vi "Write Call Chain.vi"(10 "Call Chain":string[](array[string]), 11 "Assert in":refnum<class "Assert.lvclass">) -> (3 "Assert out":refnum<class "Assert.lvclass">)   [LabVIEW 2013, in "Caraya.lvlib" / "Assert.lvclass"]
uses:
  Assert.lvclass
  Assert.lvclass/Assert.ctl
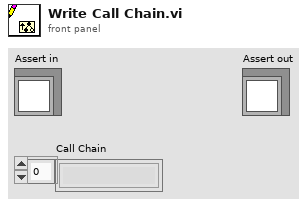
[diagram p1: front panel]
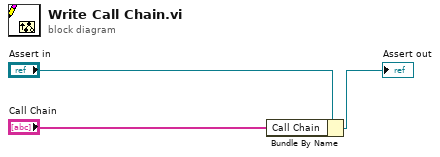
[diagram p0: block diagram]
diagram:
  n1 = Bundle By Name(cluster="Assert in", "Call Chain"="Call Chain") -> (→"Assert out":refnum<class "Assert.lvclass">)
